vi "geneXY_svi.vi"(6 "Spacing Y (µm)":dbl, 7 "Number of Positions":u32, 9 "Spacing X (µm)":dbl, 10 "Method":u8, 11 "Microscope Objective\nMagnification":dbl) -> (2 "Real Matrix":T1, 3 "field_size(µm)":dbl)   [LabVIEW 2013]
uses:
  <vilib>/Analysis/Matrix/Datatypes/RealMatrix.ctl
  <vilib>/Analysis/Matrix/Numeric/Conversions/Array To Matrix - RA.vi
  <vilib>/Analysis/Matrix/NI_Matrix.lvlib
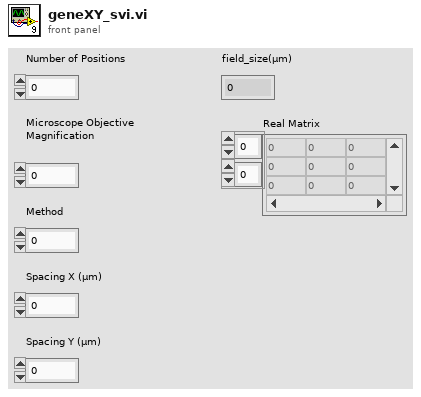
[diagram p1: front panel]
types:
  T1 = typedef "NI_Matrix.lvlib/RealMatrix.ctl" = dbl[][]
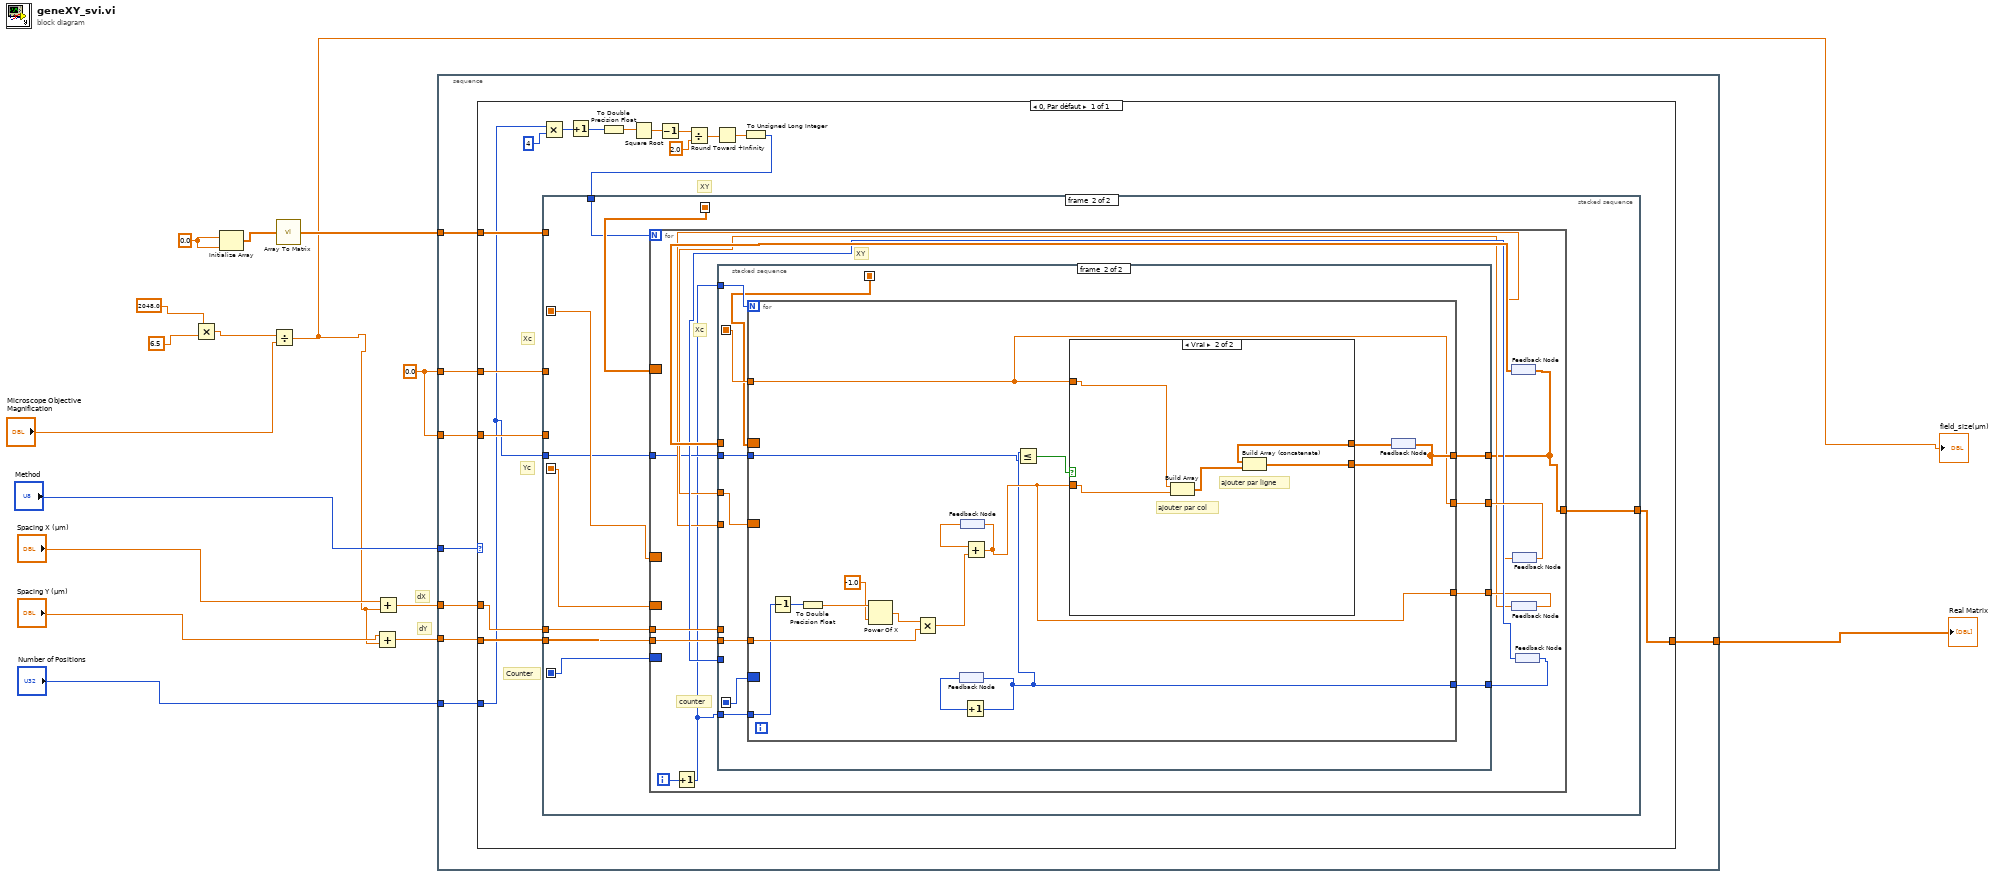
[diagram p0: block diagram]
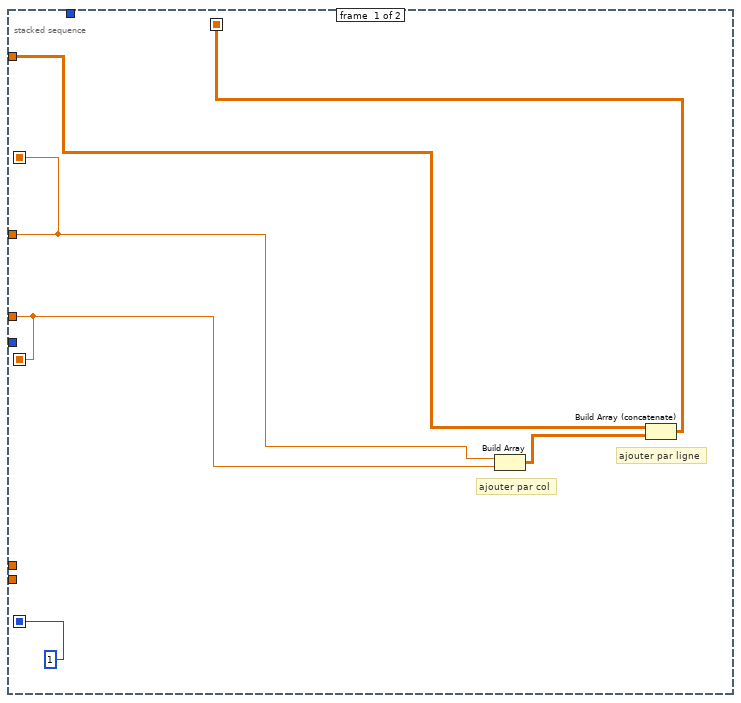
[diagram p2: hidden frame]
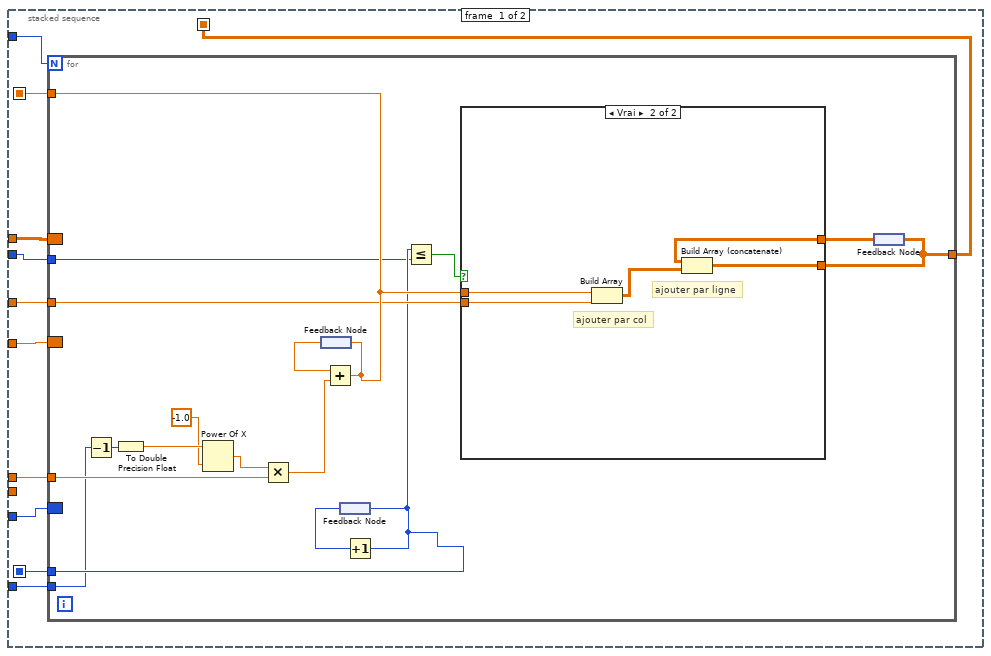
[diagram p3: hidden frame]
diagram:
  w14 = 0.0
  w12 = 0.0
  # "dY"
  # "dX"
  n1 = Multiply(x=2048.0, y=6.5) -> (x*y=w1:dbl)
  n2 = Initialize Array(w12, w12) -> (w13:dbl[])
  n3 = Divide(x=w1, y="Microscope Objective\nMagnification") -> (x/y=w2:dbl)
  "field_size(µm)" <- w2
  n4 = call-poly <vilib>:"Array To Matrix.vi"("Real 1D Array"=w13) -> ("Real Matrix (Column Vector)"=w15:T1)
  n5 = Add(x="Spacing Y (µm)", y=w2) -> (x+y=w11:dbl)
  n6 = Add(x="Spacing X (µm)", y=w2) -> (x+y=w10:dbl)
  n7 = stacked-sequence {
    tunnel: "Method" -> [w24]
    tunnel: "Number of Positions" -> [w23]
    tunnel: w10 -> [w22]
    tunnel: w11 -> [w21]
    tunnel: w14 -> [w18]
    tunnel: w14 -> [w19]
    tunnel: w15 -> [w20]
    tunnel: [w17] -> w16
    frame #0 {
      n8 = case shown="0, Par défaut" w24 {
        tunnel: w23 -> [w25]
        tunnel: w22 -> [w28]
        tunnel: w21 -> [w27]
        tunnel: w20 -> [w32]
        tunnel: w19 -> [w31]
        tunnel: w18 -> [w30]
        tunnel: [w26] -> w17
        frame 0, Default {
          # "Counter"
          # "XY"
          # "Yc"
          # "Xc"
          n9 = Multiply(x=w25, y=u32 4) -> (x*y=w41:u32)
          n10 = Increment(x=w41) -> (x+1=w39:u32)
          n11 = To Double Precision Float(number=w39) -> (double precision float=w38:dbl)
          n12 = Square Root(x=w38) -> (sqrt(x)=w37:dbl)
          n13 = Decrement(x=w37) -> (x-1=w36:dbl)
          n14 = Divide(x=w36, y=2.0) -> (x/y=w34:dbl)
          n15 = Round Toward +Infinity(x=w34) -> (ceil(x): smallest int >= x=w33:dbl)
          n16 = To Unsigned Long Integer(number=w33) -> (unsigned 32bit integer=w29:u32)
          n17 = stacked-sequence {
            seq-local: [w44 _] -> [_ w56]
            seq-local: [w46 _] -> [_ w49]
            seq-local: [w45 _] -> [_ w50]
            seq-local: [1 _] -> [_ w51]
            tunnel: w32 -> [w43 _]
            tunnel: w31 -> [w45 _]
            tunnel: w30 -> [w46 _]
            tunnel: w29 -> [_ w55]
            tunnel: [_ w54] -> w26
            tunnel: w28 -> [_ w53]
            tunnel: w27 -> [_ w52]
            tunnel: w25 -> [_ w48]
            frame #0 {
              # "ajouter par ligne"
              # "ajouter par col"
              n18 = Build Array(w46, w45) -> (w47:T1)
              n19 = Build Array (concatenate)(w43, w47) -> (w44:T1)
            }
            frame #1 {
              n20 = for {
                N: w55 -> [_]
                border: w56 -> [_]
                tunnel: [w59] -> w54
                tunnel: w53 -> [w68]
                tunnel: w52 -> [w66]
                border: w51 -> [_]
                border: w50 -> [_]
                border: w49 -> [_]
                tunnel: w48 -> [w58]
                i -> [w69]
                # "XY"
                # "counter"
                # "Xc"
                n21 = Increment(x=w69) -> (x+1=w57:i32)
                n22 = feedback #1() -> (w67:T1)
                n23 = feedback #2() -> (w60:dbl)
                n24 = feedback #3() -> (w62:dbl)
                n25 = feedback #4() -> (w63:i32)
                n26 = stacked-sequence {
                  seq-local: [w78 _] -> [_ w110]
                  seq-local: [w75 _] -> [_ w108]
                  seq-local: [w73 _] -> [_ w109]
                  tunnel: w57 -> [w80 w114]
                  tunnel: w68 -> [w79 _]
                  tunnel: w62 -> [w77 _]
                  tunnel: w63 -> [w76 _]
                  tunnel: w60 -> [w74 w111]
                  tunnel: [_ w113] -> w59
                  tunnel: w67 -> [w72 _]
                  tunnel: w66 -> [_ w112]
                  tunnel: [_ w107] -> w65
                  tunnel: [_ w106] -> w64
                  tunnel: [_ w105] -> w61
                  tunnel: w58 -> [w71 w104]
                  tunnel: w57 -> [w70 w103]
                  frame #0 {
                    n27 = for {
                      N: w80 -> [_]
                      tunnel: w79 -> [w95]
                      tunnel: [w92] -> w78
                      border: w77 -> [_]
                      border: w76 -> [_]
                      tunnel: [w87] -> w75
                      tunnel: w74 -> [w91]
                      tunnel: [w89] -> w73
                      border: w72 -> [_]
                      tunnel: w71 -> [w86]
                      tunnel: w70 -> [w82]
                      n28 = Decrement(x=w82) -> (x-1=w83:i32)
                      n29 = To Double Precision Float(number=w83) -> (double precision float=w85:dbl)
                      n30 = Power Of X(1:-1.0, 2:w85) -> (0:w96:dbl)
                      n31 = Multiply(x=w96, y=w95) -> (x*y=w81:dbl)
                      n32 = feedback #5() -> (w94:dbl)
                      n33 = Add(x=w94, y=w81) -> (x+y=w92:dbl)
                      n34 = feedback-in #5(w92) -> ()
                      n35 = feedback #6() -> (w93:i32)
                      n36 = Increment(x=w93) -> (x+1=w87:i32)
                      n37 = feedback-in #6(w87) -> ()
                      n38 = Less Or Equal?(x=w87, y=w86) -> (x <= y?=w88:bool)
                      n39 = feedback #7() -> (w90:T1)
                      n40 = case shown="Vrai" w88 {
                        tunnel: w92 -> [_ w99]
                        tunnel: w91 -> [_ w98]
                        tunnel: w90 -> [w97 w101]
                        tunnel: [w97 w100] -> w89
                        frame False {
                        }
                        frame True {
                          # "ajouter par ligne"
                          # "ajouter par col"
                          n41 = Build Array(w99, w98) -> (w102:T1)
                          n42 = Build Array (concatenate)(w101, w102) -> (w100:T1)
                        }
                      }
                      n43 = feedback-in #7(w89) -> ()
                    }
                  }
                  frame #1 {
                    n44 = for {
                      N: w114 -> [_]
                      border: w111 -> [_]
                      border: w108 -> [_]
                      tunnel: [w126] -> w113
                      tunnel: w112 -> [w125]
                      tunnel: w110 -> [w123]
                      border: w109 -> [_]
                      tunnel: [w121] -> w107
                      tunnel: [w123] -> w106
                      tunnel: [w124] -> w105
                      tunnel: w104 -> [w120]
                      tunnel: w103 -> [w116]
                      n45 = Decrement(x=w116) -> (x-1=w117:i32)
                      n46 = To Double Precision Float(number=w117) -> (double precision float=w119:dbl)
                      n47 = Power Of X(1:-1.0, 2:w119) -> (0:w130:dbl)
                      n48 = Multiply(x=w130, y=w125) -> (x*y=w115:dbl)
                      n49 = feedback #8() -> (w128:i32)
                      n50 = feedback #9() -> (w129:dbl)
                      n51 = Increment(x=w128) -> (x+1=w121:i32)
                      n52 = feedback-in #8(w121) -> ()
                      n53 = Add(x=w129, y=w115) -> (x+y=w124:dbl)
                      n54 = feedback-in #9(w124) -> ()
                      n55 = Less Or Equal?(x=w121, y=w120) -> (x <= y?=w122:bool)
                      n56 = feedback #10() -> (w127:T1)
                      n57 = case shown="Vrai" w122 {
                        tunnel: w124 -> [_ w132]
                        tunnel: w127 -> [w131 w135]
                        tunnel: [w131 w134] -> w126
                        tunnel: w123 -> [_ w133]
                        frame False {
                        }
                        frame True {
                          # "ajouter par ligne"
                          # "ajouter par col"
                          n58 = Build Array(w133, w132) -> (w136:T1)
                          n59 = Build Array (concatenate)(w135, w136) -> (w134:T1)
                        }
                      }
                      n60 = feedback-in #10(w126) -> ()
                    }
                  }
                }
                n61 = feedback-in #1(w59) -> ()
                n62 = feedback-in #2(w61) -> ()
                n63 = feedback-in #3(w64) -> ()
                n64 = feedback-in #4(w65) -> ()
              }
            }
          }
        }
      }
    }
  }
  "Real Matrix" <- w16
